vi "Resistance Test.vi"(0 "DMM ref in":refnum<visa-resource-name>, 1 "Measure\nMax Voltage":dbl=100.0, 2 "Resistance Test REF":refnum<vi>, 3 "Resistance Test Stop REF":refnum<vi>, 5 "DMM error in":errorcluster, 7 "Channel  Count":i32, 9 "ESP32 ref in":refnum<visa-resource-name>="COM4", 11 "ESP32 error in":errorcluster, 12 "Wait Current Stable Period":u32, 14 "Current Sense \nResitance Array":dbl[](array[numeric])) -> (10 "ESP32 ref out":refnum<visa-resource-name>, 15 "ESP32 error out":errorcluster)   [LabVIEW 2023]
uses:
  <instrlib>/Agilent 3446X Series/Agilent 3446X Series.lvlib
panel:
  out "Array 3":i32[][](array[numeric])
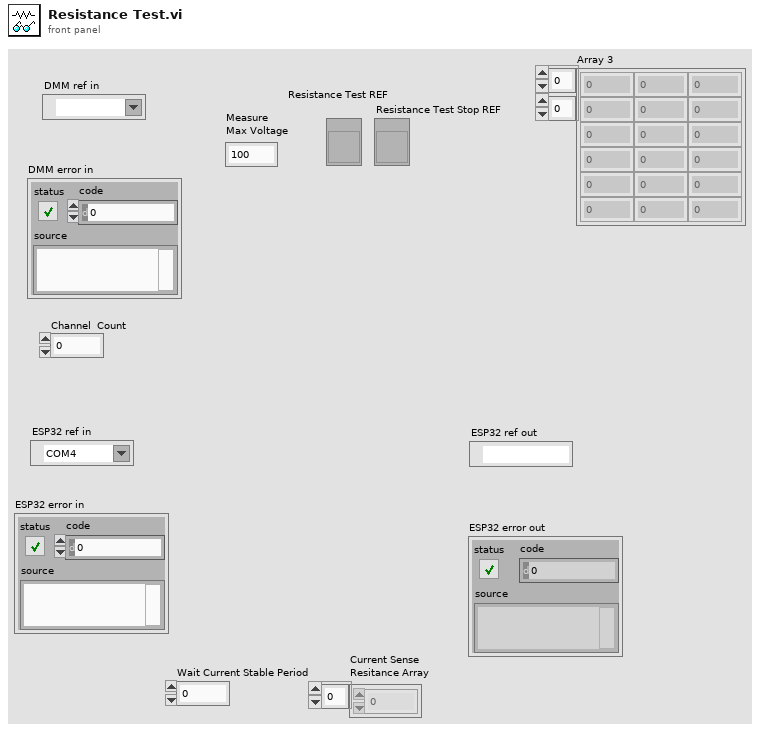
[diagram p1: front panel]
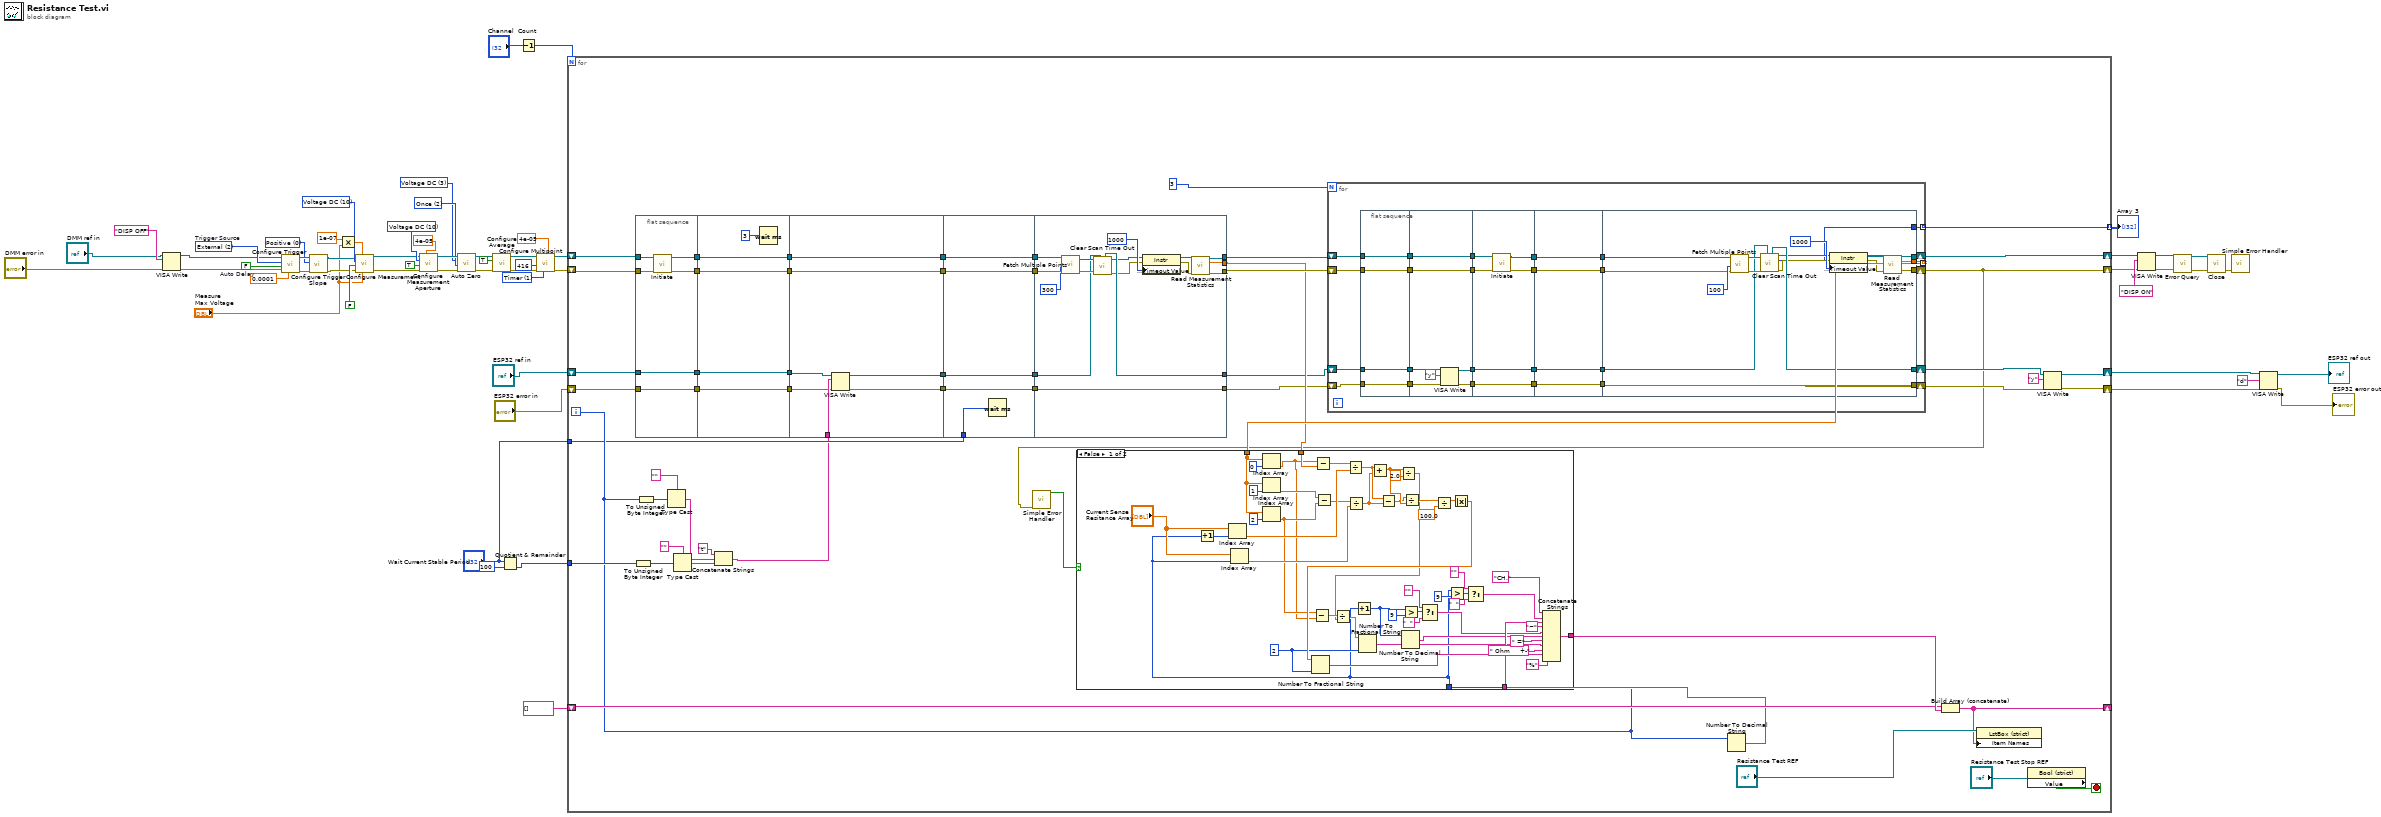
[diagram p0: block diagram]
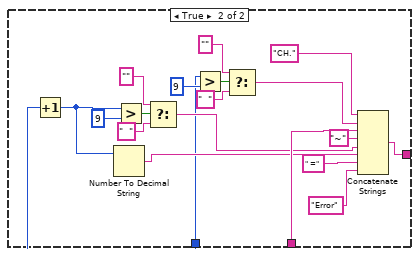
[diagram p2: hidden frame]
diagram:
  w20 = 0 items=["Positive", "Negative"] ("Trigger Edge (1: Negative)")
  w18 = 2 items=["Immediate", "Software (Bus)", "External"]  # Trigger Source
  w19 = FALSE  # Auto Delay
  w26 = 10 items=["Continuity", "Current AC", "Current DC", "Diode", "Frequency", "Resistance 4-wire", "Period", "Resistance 2-wire", "Temperature", "Voltage AC", "Voltage DC", "Voltage DC Ratio", "Capacitance"] ("Measurement Function (10: Voltage DC)")
  w30 = 1 items=["Immediate", "Timer"] ("Sample Source (0: Immediate)")
  w37 = 3 items=["Current DC", "Resistance", "Temperature", "Voltage DC"] ("Zero Type (0: Current DC)")
  w38 = 2 items=["Disable", "Enable", "Once"] ("Auto Zero (1: Enable)")
  w34 = 10 items=["Continuity", "Current AC", "Current DC", "Diode", "Frequency", "Resistance 4-wire", "Period", "Resistance 2-wire", "Temperature", "Voltage AC", "Voltage DC", "Voltage DC Ratio", "Capacitance"] ("Measurement Function (0: Continuity)")
  n1 = VISA Write(VISA resource name="DMM ref in", write buffer="DISP OFF", error in (no error)="DMM error in") -> (VISA resource name out=w3:refnum<visa-resource-name>, error out=w2:errorcluster)  [unwired: 1 out]
  n2 = call <instrlib>:"Configure Trigger.vi"("Manual Trigger Delay (1 s)"=0.0001, "error in (no error)"=w2, "Auto Delay (F:Disable)"=w19, "Trigger Source (0: Immediate)"=w18, "VISA resource name"=w3) -> ("error out"=w22:errorcluster, "VISA resource name out"=w21:refnum<visa-resource-name>)  [unwired: 1 in, 4 out]
  n3 = call <instrlib>:"Configure Trigger Slope.vi"("error in (no error)"=w22, "Trigger Edge (1: Negative)"=w20, "VISA resource name"=w21) -> ("error out"=w15:errorcluster, "VISA resource name out"=w16:refnum<visa-resource-name>)  [unwired: 7 in]
  n4 = Multiply(x=1e-07, y="Measure\nMax Voltage") -> (x*y=w27:dbl)
  n5 = call <instrlib>:"Configure Measurement.vi"("Manual Range (1)"="Measure\nMax Voltage", "Absolute Resolution (1E-6)"=w27, "error in (no error)"=w15, "Auto Range (T: Enable)"=FALSE, "Measurement Function (10: Voltage DC)"=w26, "VISA resource name"=w16) -> ("error out"=w23:errorcluster, "VISA resource name out"=w24:refnum<visa-resource-name>)  [unwired: 4 out]
  n6 = call <instrlib>:"Configure Measurement Aperture.vi"("Aperture Time (0.1s)"=4e-05, "error in (no error)"=w23, "Enable Aperture (F: Disable)"=TRUE, "Measurement Function (0: Continuity)"=w34, "VISA resource name"=w24) -> ("error out"=w41:errorcluster, "VISA resource name out"=w40:refnum<visa-resource-name>)  [unwired: 5 in]
  n7 = call <instrlib>:"Auto Zero.vi"("error in (no error)"=w41, "Auto Zero (1: Enable)"=w38, "Zero Type (0: Current DC)"=w37, "VISA resource name"=w40) -> ("error out"=w43:errorcluster, "VISA resource name out"=w42:refnum<visa-resource-name>)  [unwired: 6 in]
  n8 = call <instrlib>:"Configure Average.vi"("error in (no error)"=w43, "Enable Statistics (F: Disable)"=TRUE, "VISA resource name"=w42) -> ("error out"=w32:errorcluster, "VISA resource name out"=w33:refnum<visa-resource-name>)  [unwired: 7 in]
  n9 = Quotient & Remainder(x="Wait Current Stable Period", y=100) -> (floor(x/y)=w11:u32)  [unwired: 1 out]
  n10 = Decrement(x="Channel  Count") -> (x-1=w9:i32)
  n11 = call <instrlib>:"Configure Multipoint.vi"("Sample Interval (1 Second)"=4e-05, "Sample Source (0: Immediate)"=w30, "error in (no error)"=w32, "Sample Count (1)"=416, "VISA resource name"=w33) -> ("error out"=w13:errorcluster, "VISA resource name out"=w14:refnum<visa-resource-name>)  [unwired: 2 in, 3 out]
  n12 = for {
    N: w9 -> [_]
    shift-right: [w66] -> w45
    shift-left: "ESP32 ref in" -> [w96]
    shift-right: [w64] -> w10
    shift-left: "ESP32 error in" -> [w94]
    shift-right: [w61] -> w46
    shift-left: w13 -> [w100]
    shift-right: [w106] -> w47
    shift-left: w14 -> [w101]
    shift-right: [w108] -> _
    shift-left: string[] [] -> [w110]
    tunnel: w11 -> [w84]
    tunnel: "Wait Current Stable Period" -> [w70]
    tunnel: [w63] -> w7 mode=indexing
    i -> [w82]
    stop <- w112 stop-if-true
    n13 = To Unsigned Byte Integer(number=w84) -> (unsigned 8bit integer=w88:u8)
    n14 = flat-sequence {
      tunnel: w100 -> [w185]
      tunnel: w101 -> [w187]
      tunnel: [w186] -> w105
      tunnel: [w184] -> w104
      tunnel: [w183] -> w97
      tunnel: w96 -> [w183]
      tunnel: w94 -> [w182]
      tunnel: [w182] -> w93
      tunnel: [w192] -> w103
      tunnel: [w191] -> w102
      tunnel: w105 -> [w192]
      tunnel: w104 -> [w191]
      tunnel: w97 -> [w189]
      tunnel: [w189] -> w95
      tunnel: w93 -> [w188]
      tunnel: [w188] -> w92
      tunnel: w103 -> [w199]
      tunnel: [w199] -> w76
      tunnel: w102 -> [w198]
      tunnel: [w198] -> w78
      tunnel: w95 -> [w197]
      tunnel: w92 -> [w195]
      tunnel: w62 -> [w196]
      tunnel: [w194] -> w74
      tunnel: [w193] -> w72
      tunnel: w78 -> [w204]
      tunnel: [w204] -> w77
      tunnel: w76 -> [w203]
      tunnel: [w203] -> w75
      tunnel: w74 -> [w202]
      tunnel: [w202] -> w73
      tunnel: w72 -> [w201]
      tunnel: [w201] -> w71
      tunnel: w70 -> [w200]
      tunnel: [w217] -> w98
      tunnel: [w218] -> w99
      tunnel: w77 -> [w220]
      tunnel: w75 -> [w219]
      tunnel: [w210] -> w79
      tunnel: w73 -> [w211]
      tunnel: [w215] -> w69
      tunnel: w71 -> [w215]
      tunnel: [w214] -> w80
      frame #0 {
        n15 = call <instrlib>:"Initiate.vi"("error in (no error)"=w185, "VISA resource name"=w187) -> ("error out"=w184:errorcluster, "VISA resource name out"=w186:refnum<visa-resource-name>)  [unwired: 8 out]
      }
      frame #1 {
        n16 = Wait (ms)(milliseconds to wait=u32 3) -> ()  [unwired: 1 out]
      }
      frame #2 {
        n17 = VISA Write(VISA resource name=w197, write buffer=w196, error in (no error)=w195) -> (VISA resource name out=w194:refnum<visa-resource-name>, error out=w193:errorcluster)  [unwired: 1 out]
      }
      frame #3 {
        n18 = Wait (ms)(milliseconds to wait=w200) -> ()  [unwired: 1 out]
      }
      frame #4 {
        n19 = call <instrlib>:"Fetch Multiple Points.vi"("error in (no error)"=w220, "Timeout (10000 ms)"=300, "VISA resource name"=w219) -> ("error out"=w212:errorcluster, "VISA resource name out"=w213:refnum<visa-resource-name>)  [unwired: 1 in, 6 out]
        n20 = call "Clear Scan Time Out.vi"("ESP32 ref"=w211, "error in (no error)"=w212, "VISA Refnum in"=w213) -> ("error out"=w207:errorcluster, "VISA Refnum out"=w208:refnum<visa-resource-name>, "ESP32 ref out"=w210:refnum<visa-resource-name>)  [unwired: 4 in, 2 out]
        n21 = property class="Instr"(reference=w208, error in=w207, "General Settings:Timeout Value"=u32 1000) -> (reference out=w206:refnum<visa-resource-name>, error out=w205:errorcluster)
        n22 = call <instrlib>:"Read Measurement Statistics.vi"("VISA resource name"=w206, "error in (no error)"=w205) -> ("VISA resource name out"=w218:refnum<visa-resource-name>, "Arithmetic Mean"=w214:dbl, "error out"=w217:errorcluster)  [unwired: 6 in, 5 out]
      }
    }
    n23 = To Unsigned Byte Integer(number=w82) -> (unsigned 8bit integer=w85:u8)
    n24 = Type Cast(type="" ("string"), x=w85) -> (*(type *) &x=w86:string)
    n25 = Type Cast(type="" ("string"), x=w88) -> (*(type *) &x=w87:string)
    n26 = Concatenate Strings("t" ("data in"), w86, w87) -> (w62:string)
    n27 = for {
      N: 3 -> [_]
      tunnel: [w244] -> w81 mode=indexing
      shift-right: [w243] -> w106
      shift-left: w99 -> [w246]
      shift-right: [w242] -> w61
      shift-left: w98 -> [w245]
      shift-right: [w240] -> w67
      shift-left: w79 -> [w241]
      shift-right: [w238] -> w65
      shift-left: w69 -> [w239]
      tunnel: [w237] -> w63 mode=indexing
      n28 = flat-sequence {
        tunnel: w239 -> [w247]
        tunnel: w241 -> [w248]
        tunnel: w245 -> [w249]
        tunnel: w246 -> [w250]
        tunnel: [w250] -> w236
        tunnel: [w249] -> w235
        tunnel: [w248] -> w234
        tunnel: [w247] -> w233
        tunnel: [w257] -> w232
        tunnel: [w256] -> w231
        tunnel: [w254] -> w230
        tunnel: [w251] -> w229
        tunnel: w236 -> [w257]
        tunnel: w235 -> [w256]
        tunnel: w234 -> [w255]
        tunnel: w233 -> [w252]
        tunnel: w232 -> [w261]
        tunnel: w231 -> [w260]
        tunnel: [w259] -> w228
        tunnel: w230 -> [w263]
        tunnel: [w263] -> w226
        tunnel: w229 -> [w262]
        tunnel: [w262] -> w224
        tunnel: [w258] -> w222
        tunnel: w228 -> [w267]
        tunnel: [w267] -> w227
        tunnel: w226 -> [w266]
        tunnel: [w266] -> w225
        tunnel: w224 -> [w265]
        tunnel: [w265] -> w223
        tunnel: w222 -> [w264]
        tunnel: [w264] -> w221
        tunnel: [w284] -> w244
        tunnel: [w282] -> w243
        tunnel: [w281] -> w242
        tunnel: [w277] -> w240
        tunnel: w227 -> [w268]
        tunnel: w225 -> [w278]
        tunnel: w223 -> [w271]
        tunnel: [w271] -> w238
        tunnel: [w270] -> w237
        tunnel: w221 -> [w269]
        frame #0 {
        }
        frame #1 {
          n29 = VISA Write(VISA resource name=w255, write buffer="y", error in (no error)=w252) -> (VISA resource name out=w254:refnum<visa-resource-name>, error out=w251:errorcluster)  [unwired: 1 out]
        }
        frame #2 {
          n30 = call <instrlib>:"Initiate.vi"("error in (no error)"=w260, "VISA resource name"=w261) -> ("error out"=w259:errorcluster, "VISA resource name out"=w258:refnum<visa-resource-name>)  [unwired: 8 out]
        }
        frame #3 {
        }
        frame #4 {
          n31 = call <instrlib>:"Fetch Multiple Points.vi"("error in (no error)"=w268, "Timeout (10000 ms)"=100, "VISA resource name"=w269) -> ("error out"=w279:errorcluster, "VISA resource name out"=w280:refnum<visa-resource-name>)  [unwired: 1 in, 6 out]
          n32 = call "Clear Scan Time Out.vi"("ESP32 ref"=w278, "error in (no error)"=w279, "VISA Refnum in"=w280) -> ("error out"=w272:errorcluster, "Time out count"=w270:i32, "VISA Refnum out"=w273:refnum<visa-resource-name>, "ESP32 ref out"=w277:refnum<visa-resource-name>)  [unwired: 4 in, 1 out]
          n33 = property class="Instr"(reference=w273, error in=w272, "General Settings:Timeout Value"=u32 1000) -> (reference out=w275:refnum<visa-resource-name>, error out=w274:errorcluster)
          n34 = call <instrlib>:"Read Measurement Statistics.vi"("VISA resource name"=w275, "error in (no error)"=w274) -> ("VISA resource name out"=w282:refnum<visa-resource-name>, "Arithmetic Mean"=w284:dbl, "error out"=w281:errorcluster)  [unwired: 6 in, 5 out]
        }
      }
    }
    n35 = call <vilib>:"Simple Error Handler.vi"("error in (no error)"=w61) -> ("error?"=w60:bool)  [unwired: 4 in, 4 out]
    n36 = Number To Decimal String(number=w82) -> (decimal integer string=w83:string)  [unwired: 1 in]
    n37 = case shown="False" w60 {
      tunnel: [w157 w176] -> w111
      tunnel: w83 -> [w154 w173]
      tunnel: w81 -> [w142 _]
      tunnel: w82 -> [w118 w164]
      tunnel: w80 -> [w135 _]
      frame False {
        w126 = i16 2 ("precision (6)")
        n38 = Increment(x=w118) -> (x+1=w138:i32)
        n39 = Index Array(array="Current Sense \nResitance Array", index=w138) -> (element=w136:dbl)
        n40 = Index Array(array="Current Sense \nResitance Array", index=w118) -> (element=w133:dbl)
        n41 = Index Array(array=w142, index=0) -> (element=w122:dbl)
        n42 = Index Array(array=w142, index=1) -> (element=w123:dbl)
        n43 = Index Array(array=w142, index=2) -> (element=w124:dbl)
        n44 = Subtract(x=w124, y=w122) -> (x-y=w121:dbl)
        n45 = Subtract(x=w122, y=w135) -> (x-y=w139:dbl)
        n46 = Subtract(x=w123, y=w124) -> (x-y=w134:dbl)
        n47 = Divide(x=w139, y=w136) -> (x/y=w131:dbl)
        n48 = Divide(x=w134, y=w133) -> (x/y=w130:dbl)
        n49 = Increment(x=w118) -> (x+1=w147:i32)
        n50 = Add(x=w131, y=w130) -> (x+y=w117:dbl)
        n51 = Subtract(x=w131, y=w130) -> (x-y=w116:dbl)
        n52 = Divide(x=w117, y=2.0) -> (x/y=w120:dbl)
        n53 = Divide(x=w121, y=w120) -> (x/y=w119:dbl)
        n54 = Number To Fractional String(number=w119, precision (6)=w126) -> (F-format string=w128:string)  [unwired: 2 in]
        n55 = Number To Decimal String(number=w147) -> (decimal integer string=w146:string)  [unwired: 1 in]
        n56 = Greater?(x=w147, y=9) -> (0:w151:bool)
        n57 = Divide(x=w116, y=w117) -> (x/y=w129:dbl)
        n58 = Select(t="" ("string"), s=w151, f="  " ("string")) -> (s? t:f=w148:string)
        n59 = Divide(x=w129, y=100.0) -> (x/y=w115:dbl)
        n60 = Greater?(x=w118, y=9) -> (0:w160:bool)
        n61 = Absolute Value(x=w115) -> (abs(x)=w127:dbl)
        n62 = Number To Fractional String(number=w127, precision (6)=w126) -> (F-format string=w125:string)  [unwired: 2 in]
        n63 = Select(t="" ("string"), s=w160, f="  " ("string")) -> (s? t:f=w155:string)
        n64 = Concatenate Strings("CH." ("string"), w155, w154, "~" ("string"), w148, w146, " =" ("string"), w128, " Ohm     +-" ("string"), w125, "%" ("string")) -> (w157:string)
      }
      frame True {
        n65 = Increment(x=w164) -> (x+1=w166:i32)
        n66 = Number To Decimal String(number=w166) -> (decimal integer string=w165:string)  [unwired: 1 in]
        n67 = Greater?(x=w166, y=9) -> (0:w170:bool)
        n68 = Select(t="" ("string"), s=w170, f="  " ("string")) -> (s? t:f=w167:string)
        n69 = Greater?(x=w164, y=9) -> (0:w179:bool)
        n70 = Select(t="" ("string"), s=w179, f="  " ("string")) -> (s? t:f=w174:string)
        n71 = Concatenate Strings("CH." ("string"), w174, w173, "~" ("string"), w167, w165, " =" ("string"), "Error" ("string")) -> (w176:string)
      }
    }
    n72 = Build Array (concatenate)(w110, w111) -> (w108:string[])
    n73 = property class="LstBox (strict)"(reference="Resistance Test REF", "Item Names"=w108) -> ()  [unwired: 1 in, 2 out]
    n74 = property class="Bool (strict)"(reference="Resistance Test Stop REF") -> ("Value"=w112:bool)  [unwired: 1 in, 2 out]
    n75 = VISA Write(VISA resource name=w67, write buffer="y", error in (no error)=w65) -> (VISA resource name out=w66:refnum<visa-resource-name>, error out=w64:errorcluster)  [unwired: 1 out]
  }
  "Array 3" <- w7
  n76 = VISA Write(VISA resource name=w47, write buffer="DISP ON", error in (no error)=w46) -> (VISA resource name out=w54:refnum<visa-resource-name>, error out=w53:errorcluster)  [unwired: 1 out]
  n77 = call <instrlib>:"Error Query.vi"("error in (no error)"=w53, "VISA resource name"=w54) -> ("error out"=w59:errorcluster, "VISA resource name out"=w58:refnum<visa-resource-name>)  [unwired: 8 out]
  n78 = call <instrlib>:"Close.vi"("error in (no error)"=w59, "VISA resource name"=w58) -> ("error out"=w57:errorcluster)  [unwired: 9 out]
  n79 = call <vilib>:"Simple Error Handler.vi"("error in (no error)"=w57) -> ()  [unwired: 1 in, 8 out]
  n80 = VISA Write(VISA resource name=w45, write buffer="d" ("data in"), error in (no error)=w10) -> (VISA resource name out=→"ESP32 ref out":refnum<visa-resource-name>, error out=→"ESP32 error out":errorcluster)  [unwired: 1 out]
